vi "UIRef.vi"(8 "error in":errorcluster, 11 "tag select module editor node in":refnum<class "tag select module editor node.lvclass">) -> (0 "error out":errorcluster, 2 "VI refnum":refnum<vi>, 3 "tag select module editor node out":refnum<class "tag select module editor node.lvclass">)   [LabVIEW 2015, in "tag select module editor node.lvclass"]
uses:
  tag select module editor node.lvclass
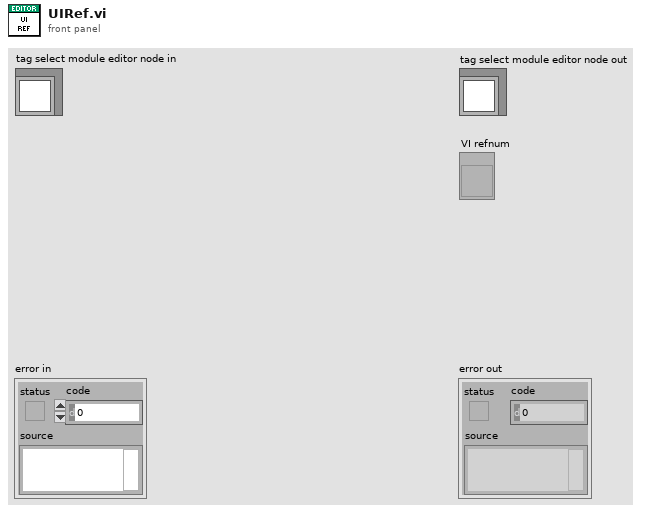
[diagram p1: front panel]
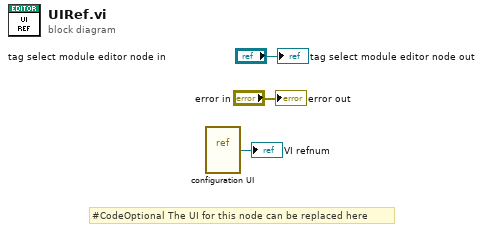
[diagram p0: block diagram]
diagram:
  # "#CodeOptional The UI for this node can be replaced here"
  n1 = vi-ref "configuration UI.vi"() -> (→"VI refnum":refnum<vi>)
  "error out" <- "error in"
  "tag select module editor node out" <- "tag select module editor node in"
